vi "read.vi"(6 "timeout (0)":i32, 8 "error in (no error)":errorcluster, 9 "bufferSize":i64, 11 "IStreamReader in":refnum<class "IStreamReader.lvclass">) -> (0 "error out":errorcluster, 1 "Reader Status out":refnum<class "IReaderStatus.lvclass">, 2 "Read Buffers out":dbl[](array[numeric]), 3 "IStreamReader out":refnum<class "IStreamReader.lvclass">)   [LabVIEW 2022 SP3, in "openDAQ.lvlib" / "IBaseObject.lvlib" / "IReader.lvlib" / "ISampleReader.lvlib" / "IStreamReader.lvlib" / "IStreamReader.lvclass"]
uses:
  <instrlib>/openDAQ/Public/Classes/IStreamReader/IStreamReader.lvclass
  C:/Program Files (x86)/National Instruments/LabVIEW 2022/instr.lib/openDAQ/Public/Classes/IBaseObject/IBaseObject.lvclass
  <instrlib>/openDAQ/Public/Classes/IReaderStatus/IReaderStatus.lvclass
  <instrlib>/openDAQ/Public/Classes/IMultiReaderStatus/IMultiReaderStatus.lvclass
  C:/Program Files (x86)/National Instruments/LabVIEW 2022/instr.lib/openDAQ/Public/Classes/IReaderStatus/IReaderStatus.lvclass
  <instrlib>/openDAQ/Public/Classes/IBaseObject/IBaseObject.lvclass/IBaseObject.ctl
  <instrlib>/openDAQ/Public/Classes/IBaseObject/Accessor/Read reference.vi
  <instrlib>/openDAQ/Public/Classes/IBaseObject/Accessor/Write reference.vi
  <instrlib>/openDAQ/Public/Classes/IStreamReader/IStreamReader.lvclass/IStreamReader.ctl
  <instrlib>/openDAQ/Binaries/Windows/x86/copendaq32.dll
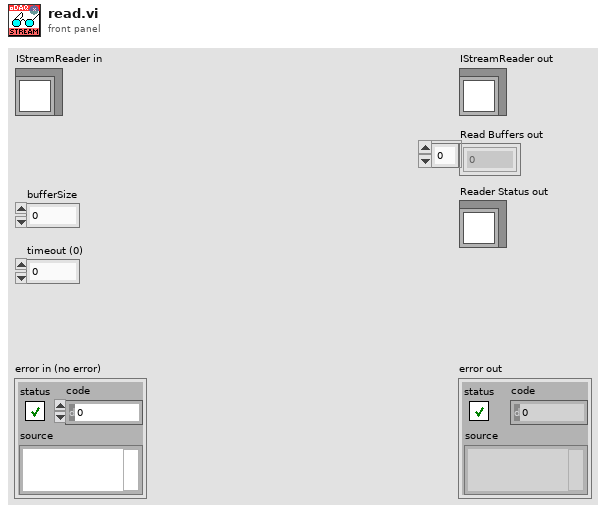
[diagram p1: front panel]
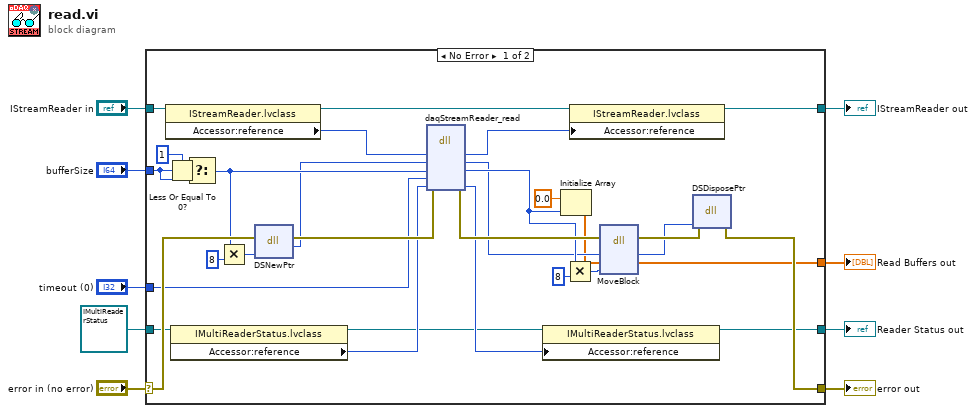
[diagram p0: block diagram]
diagram:
  n1 = case shown="No Error" "error in (no error)" {
    selector: "error in (no error)" -> [w37 w43]
    tunnel: [w40 w43] -> w8
    tunnel: [w34 w42] -> w6
    tunnel: "IStreamReader in" -> [w36 w42]
    tunnel: "bufferSize" -> [w23 _]
    tunnel: refnum<class "IMultiReaderStatus.lvclass"> refnum ("openDAQ.lvlib:IBaseObject.lvlib:IReaderStatus.lvlib:IMultiReaderStatus.lvlib:IMultiReaderStatus.lvclass") -> [w31 w41]
    tunnel: [w27 w41] -> w3
    tunnel: "timeout (0)" -> [w26 _]
    tunnel: [w19 _] -> w1
    frame No Error {
      n2 = property class="IStreamReader.lvclass"(reference=w36) -> (reference out=w35:refnum<class "IStreamReader.lvclass">, "Accessor:reference"=w33:i64)  [unwired: 1 in, 1 out]
      n3 = Less Or Equal To 0?(x=w23) -> (x <= 0?=w25:bool)
      n4 = property class="IMultiReaderStatus.lvclass"(reference=w31) -> (reference out=w28:refnum<class "IMultiReaderStatus.lvclass">, "Accessor:reference"=w30:i64)  [unwired: 1 in, 1 out]
      n5 = Select(t=i64 1, s=w25, f=w23) -> (s? t:f=w24:i64)
      n6 = Multiply(x=w24, y=i64 8) -> (x*y=w17:i64)
      n7 = dll-call lib="LabVIEW" fn="DSNewPtr"(error in=w37, "size"=w17) -> (error out=w38:errorcluster, "block*"=w16:i64)  [unwired: 3 in, 1 out]
      n8 = dll-call lib="C:/Program Files (x86)/National Instruments/LabVIEW 2022/instr.lib/openDAQ/Binaries/Windows/x86/copendaq*.*" fn="daqStreamReader_read"(error in=w38, "streamReader"=w33, "dataBuffers"=w16, "count"=w24, "timeout"=w26, "status"=w30) -> (error out=w39:errorcluster, "streamReader"=w32:i64, "dataBuffers"=w20:i64, "count"=w21:i64, "status"=w29:i64)  [unwired: 4 in, 1 out]
      n9 = property class="IMultiReaderStatus.lvclass"(reference=w28, "Accessor:reference"=w29) -> (reference out=w27:refnum<class "IMultiReaderStatus.lvclass">)  [unwired: 1 in, 1 out]
      n10 = Initialize Array(0.0 ("element"), w21) -> (w12:dbl[])
      n11 = Multiply(x=w21, y=i64 8) -> (x*y=w14:i64)
      n12 = property class="IStreamReader.lvclass"(reference=w35, "Accessor:reference"=w32) -> (reference out=w34:refnum<class "IStreamReader.lvclass">)  [unwired: 1 in, 1 out]
      n13 = dll-call lib="LabVIEW" fn="MoveBlock"(error in=w39, "start"=w20, "destination"=w12, "size"=w14) -> (error out=w11:errorcluster, "start"=w10:i64, "destination"=w19:dbl[])  [unwired: 4 in, 1 out]
      n14 = dll-call lib="LabVIEW" fn="DSDisposePtr"(error in=w11, "pointer"=w10) -> (error out=w40:errorcluster)  [unwired: 4 in, 1 out]
    }
    frame Error {
    }
  }
  "error out" <- w8
  "IStreamReader out" <- w6
  "Reader Status out" <- w3
  "Read Buffers out" <- w1
